vi "Problem 6 - Sum square difference.vi"() -> (2 "Execution time (ms)":u32, 3 "Answer":i32)   [LabVIEW 2021, in "Project Euler.lvlib"]
uses:
  Project Euler.lvlib
  Utilities/Named Timers/Named Timers.lvlib
panel:
  # "Development\nControls or indicators that are useful for development or testing, but which are not outputs of the VI."
  # "Input\nInputs to the VI"
  # "Output\nOutputs of the VI"
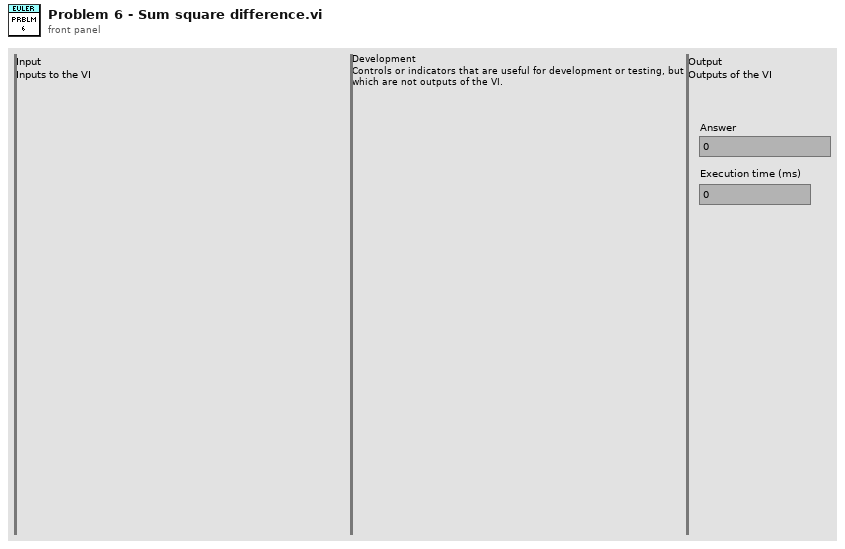
[diagram p1: front panel]
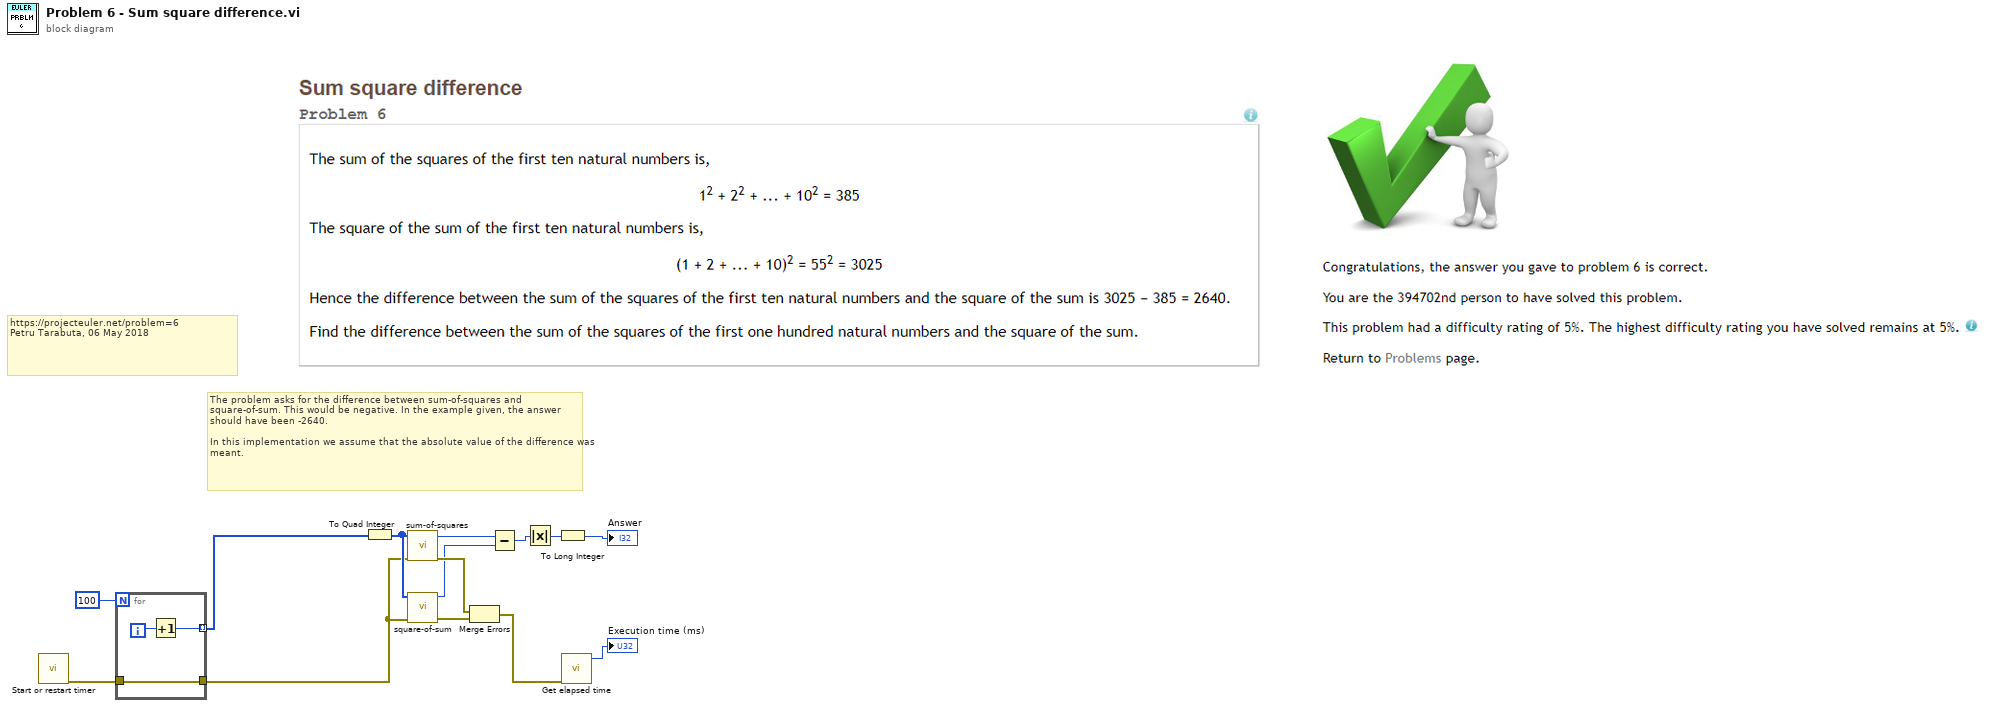
[diagram p0: block diagram]
diagram:
  # "The problem asks for the difference between sum-of-squares and square-of-sum. This would be negative. In the example given, the answer should have been -2640.\n\nIn this implementation we assume that the absolute value of the difference was meant."
  # "https://projecteuler.net/problem=6\nPetru Tarabuta, 06 May 2018"
  n1 = call "Start or restart timer.vi"() -> ("error out"=w10:errorcluster)  [unwired: 11 in]
  n2 = for {
    N: 100 -> [_]
    tunnel: [w16] -> w12 mode=indexing
    tunnel: w10 -> [w15]
    tunnel: [w15] -> w9
    i -> [w17]
    n3 = Increment(x=w17) -> (x+1=w16:i32)
  }
  n4 = To Quad Integer(1:w12) -> (0:w11:i64[])
  n5 = call "sum-of-squares.vi"("error in (no error)"=w9, "Input integers"=w11) -> ("error out"=w8:errorcluster, "sum-of-squares"=w5:i64)  [unwired: 8 in]
  n6 = call "square-of-sum.vi"("error in (no error)"=w9, "Input integers"=w11) -> ("error out"=w7:errorcluster, "square-of-sum"=w4:i64)  [unwired: 8 in]
  n7 = Merge Errors(w8, w7) -> (w6:errorcluster)
  n8 = Subtract(x=w5, y=w4) -> (x-y=w3:i64)
  n9 = Absolute Value(x=w3) -> (abs(x)=w2:i64)
  n10 = To Long Integer(number=w2) -> (32bit integer=→"Answer":i32)
  n11 = call "Get elapsed time.vi"("error in (no error)"=w6) -> ("Elapsed time (ms)"=→"Execution time (ms)":u32)  [unwired: 7 in, 3 out]
